vi "Update From Typedef.vi"(11 "VI references":refnum<vi>[](array[refnum])) -> ()   [LabVIEW 2014, in "control module data interface generator.lvlib"]
uses:
  control module data interface generator.lvlib
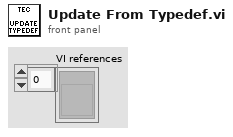
[diagram p1: front panel]
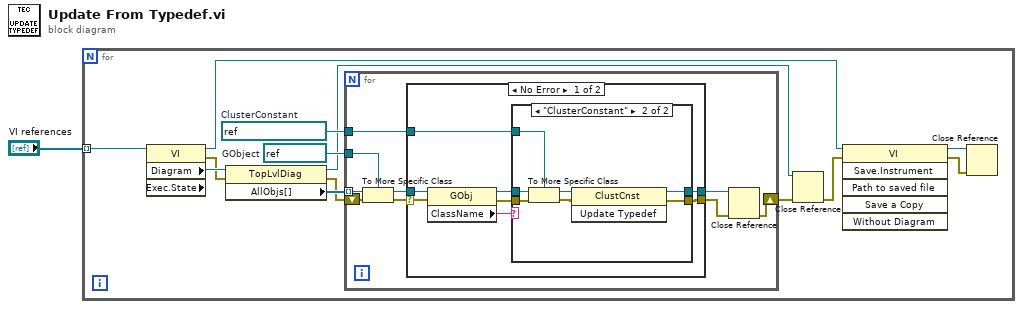
[diagram p0: block diagram]
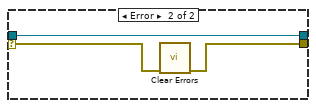
[diagram p3: hidden frame]
diagram:
  n1 = for {
    tunnel: "VI references" -> [w2] mode=indexing
    w7 = refnum<vi> refnum  # ClusterConstant
    w8 = refnum<vi> refnum  # GObject
    n2 = property class="VI" props=["Diagram", "Exec.State"](reference=w2) -> (reference out=w3:refnum<vi>, error out=w11:errorcluster, "Diagram"=w12:refnum<vi>)  [unwired: 1 in, 1 out]
    n3 = property class="TopLvlDiag"(reference=w12, error in=w11) -> (reference out=w6:refnum<vi>, error out=w9:errorcluster, "AllObjs[]"=w10:refnum<vi>[])
    n4 = for {
      tunnel: w10 -> [w23] mode=indexing
      tunnel: w8 -> [w19]
      tunnel: w7 -> [w18]
      shift-right: [w16] -> w4
      shift-left: w9 -> [w22]
      n5 = To More Specific Class(target class=w19, reference=w23, error in=w22) -> (specific class reference=w20:refnum<vi>, error out=w21:errorcluster)
      n6 = case shown="No Error" w21 {
        selector: w21 -> [w30 w42]
        tunnel: w20 -> [w31 w43]
        tunnel: [w26 w43] -> w17
        tunnel: [w25 w41] -> w15
        tunnel: w18 -> [w24 _]
        frame No Error {
          n7 = property class="GObj"(reference=w31, error in=w30) -> (reference out=w28:refnum<vi>, error out=w27:errorcluster, "ClassName"=w29:string)
          n8 = case shown="\"ClusterConstant\"" w29 {
            tunnel: w28 -> [w33 w38]
            tunnel: w27 -> [w32 w37]
            tunnel: [w33 w40] -> w26
            tunnel: [w32 w39] -> w25
            tunnel: w24 -> [_ w34]
            frame Default {
            }
            frame "ClusterConstant" {
              n9 = To More Specific Class(target class=w34, reference=w38, error in=w37) -> (specific class reference=w35:refnum<vi>, error out=w36:errorcluster)
              n10 = invoke class="ClustCnst" method="Update Typedef"(reference=w35, error in=w36) -> (reference out=w40:refnum<vi>, error out=w39:errorcluster)  [unwired: 1 in, 1 out]
            }
          }
        }
        frame Error {
          n11 = call <vilib>:"Clear Errors.vi"("error in (no error)"=w42) -> ("error out"=w41:errorcluster)  [unwired: 5 in, 1 out]
        }
      }
      n12 = Close Reference(reference=w17, error in (no error)=w15) -> (error out=w16:errorcluster)
    }
    n13 = Close Reference(reference=w6, error in (no error)=w4) -> (error out=w5:errorcluster)
    n14 = invoke class="VI" method="Save.Instrument"(reference=w3, error in=w5) -> (reference out=w14:refnum<vi>, error out=w13:errorcluster)  [unwired: 4 in, 4 out]
    n15 = Close Reference(reference=w14, error in (no error)=w13) -> ()  [unwired: 1 out]
  }
